vi "UpperCaseLowerCase.vi"() -> ()   [LabVIEW 2019]
panel:
  out "Lowerstr3":string
  out "Lowerstr2":string
  out "Upperstr1":string
  in  "str3":string="Hello"
  in  "str2":string="HELLO"
  in  "str1":string="hello"
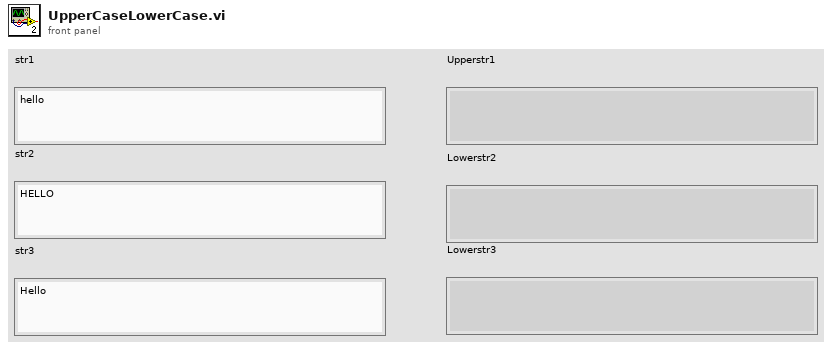
[diagram p1: front panel]
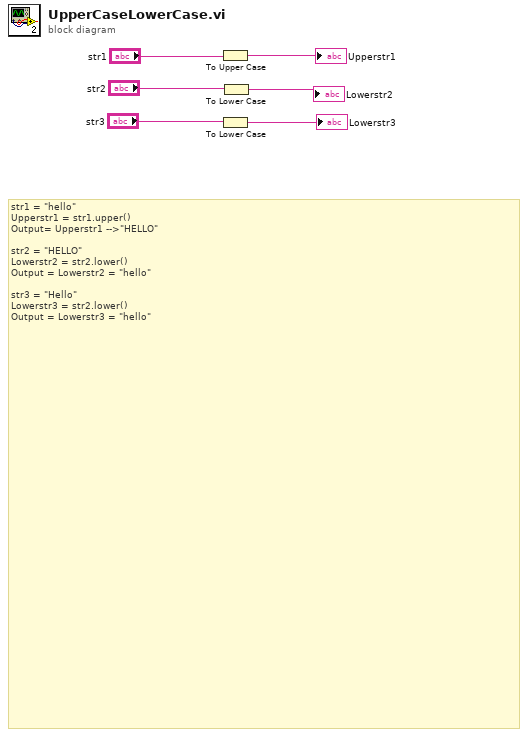
[diagram p0: block diagram]
diagram:
  # "str1 = \"hello\"\nUpperstr1 = str1.upper()\nOutput= Upperstr1 -->\"HELLO\"\n\nstr2 = \"HELLO\"\nLowerstr2 = str2.lower()\nOutput = Lowerstr2 = \"hello\"\n\nstr3 = \"Hello\"\nLowerstr3 = str2.lower()\nOutput = Lowerstr3 = \"hello\""
  n1 = To Upper Case(1:"str1") -> (0:→"Upperstr1":string)
  n2 = To Lower Case(string="str3") -> (all lower case string=→"Lowerstr3":string)
  n3 = To Lower Case(string="str2") -> (all lower case string=→"Lowerstr2":string)
